vi "1-17.vi"() -> ()   [LabVIEW 2022 SP3]
panel:
  out "循环次数":dbl
  out "随机数":dbl
  in  "指定数值":dbl
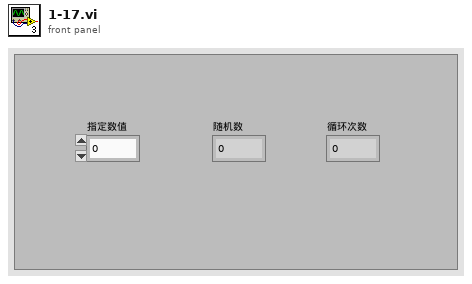
[diagram p1: front panel]
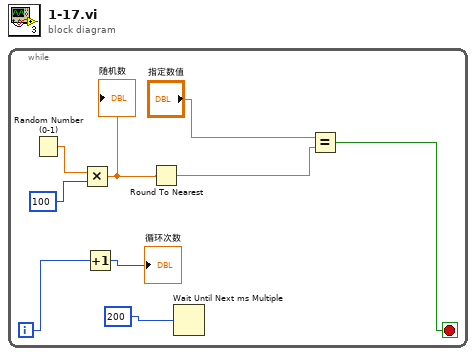
[diagram p0: block diagram]
diagram:
  n1 = while {
    i -> [w9]
    stop <- w1 stop-if-true
    n2 = Random Number (0-1)() -> (number: 0 to 1=w6:dbl)
    n3 = Multiply(x=w6, y=100) -> (x*y=w3:dbl)
    "随机数" <- w3
    n4 = Increment(x=w9) -> (x+1=→"循环次数":i32)
    n5 = Round To Nearest(number=w3) -> (nearest integer value=w2:dbl)
    n6 = Wait Until Next ms Multiple(millisecond multiple=200) -> ()  [unwired: 1 out]
    n7 = Equal?(x="指定数值", y=w2) -> (x = y?=w1:bool)
  }
